vi "Calculate Vertex Array.vi"(8 "error in (no error)":errorcluster, 9 "Coordinates System":enum16{"Cartesian", "Cylindrical", "Spherical"}(ring)=enum."Spherical", 10 "3D Waterfall Datatype.lvclass in":refnum<class "3D Waterfall Datatype.lvclass">, 11 "Plot Representation In":T1) -> (0 "error out":errorcluster, 1 "Dup Coordinates System":enum16{"Cartesian", "Cylindrical", "Spherical"}(ring)=enum."Spherical", 2 "3D Waterfall Datatype.lvclass out":refnum<class "3D Waterfall Datatype.lvclass">, 3 "Plot Representation Out":T1)   [LabVIEW 2020, in "3D Waterfall Datatype.lvclass"]
uses:
  <vilib>/Math Plots/3D Math Plots/3D Waterfall/3D Waterfall Datatype/3D Waterfall Datatype.lvclass
  <vilib>/Math Plots/3D Math Plots/3D Plot/3D Plot/Typedef/Plot Representation.ctl
  <vilib>/Math Plots/3D Math Plots/3D Plot/3D Plot/Typedef/Range Clusters.ctl
  <vilib>/Math Plots/3D Math Plots/3D Plot/3D Plot/Typedef/Mesh Data.ctl
  <vilib>/Math Plots/3D Math Plots/3D Waterfall/3D Waterfall Datatype/3D Waterfall Datatype.lvclass/3D Waterfall Datatype.ctl
  <vilib>/Math Plots/3D Math Plots/3D Plot/3D Plot Datatype/3D Plot Datatype.lvclass
  <vilib>/Math Plots/3D Math Plots/3D Plot/3D Plot/3D Plot.lvclass
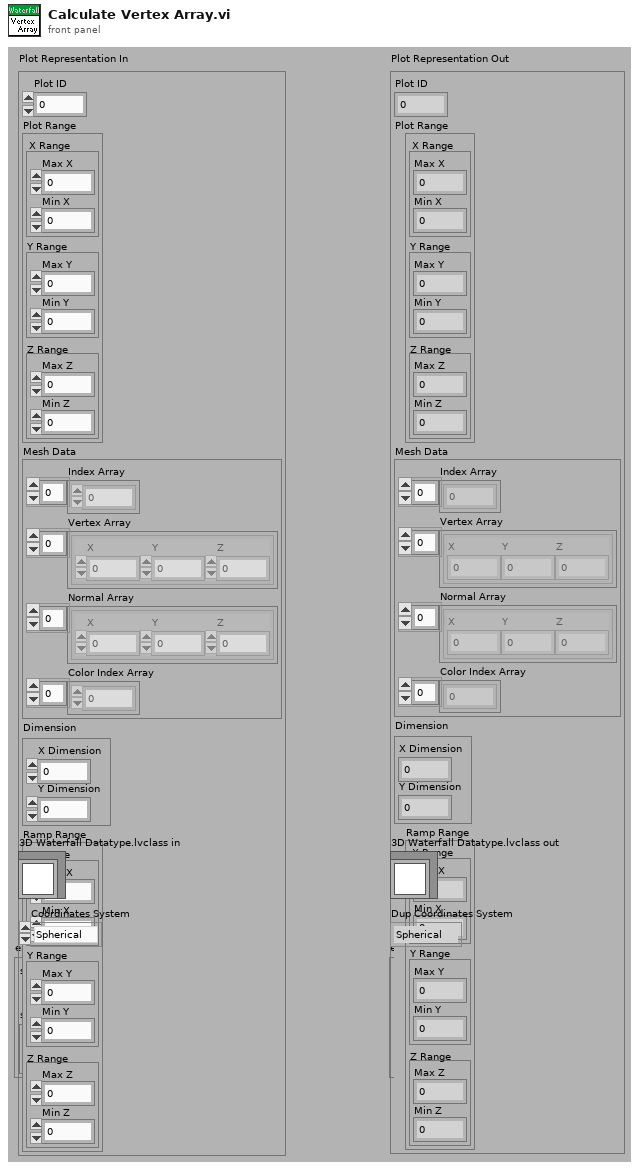
[diagram p1: front panel]
types:
  T1 = typedef "3D Plot.lvclass/Plot Representation.ctl" = cluster{"Plot ID":i32, "Plot Range":T2, "Mesh Data":T3, "Dimension":cluster{"X Dimension":i32, "Y Dimension":i32}, "Ramp Range":T2}
  T2 = typedef "3D Plot.lvclass/Range Clusters.ctl" = cluster{"X Range":cluster{"Max X":sgl, "Min X":sgl}, "Y Range":cluster{"Max Y":sgl, "Min Y":sgl}, "Z Range":cluster{"Max Z":sgl, "Min Z":sgl}}
  T3 = typedef "3D Plot.lvclass/Mesh Data.ctl" = cluster{"Index Array":u32[], "Vertex Array":cluster{"X":sgl, "Y":sgl, "Z":sgl}[], "Normal Array":cluster{"X":sgl, "Y":sgl, "Z":sgl}[], "Color Index Array":i32[]}
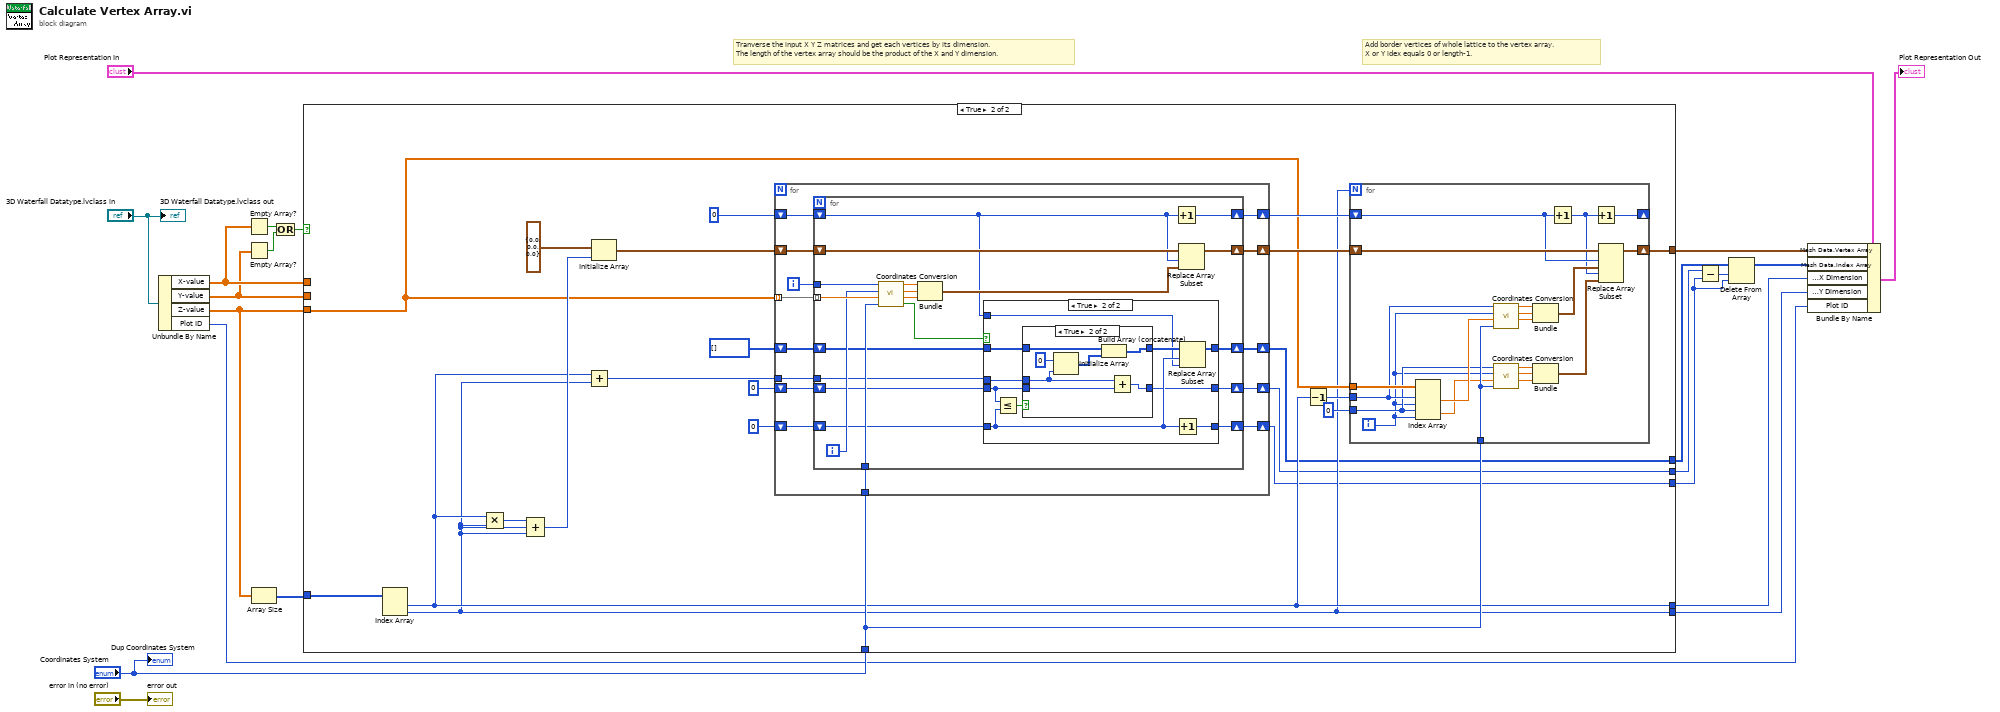
[diagram p0: block diagram]
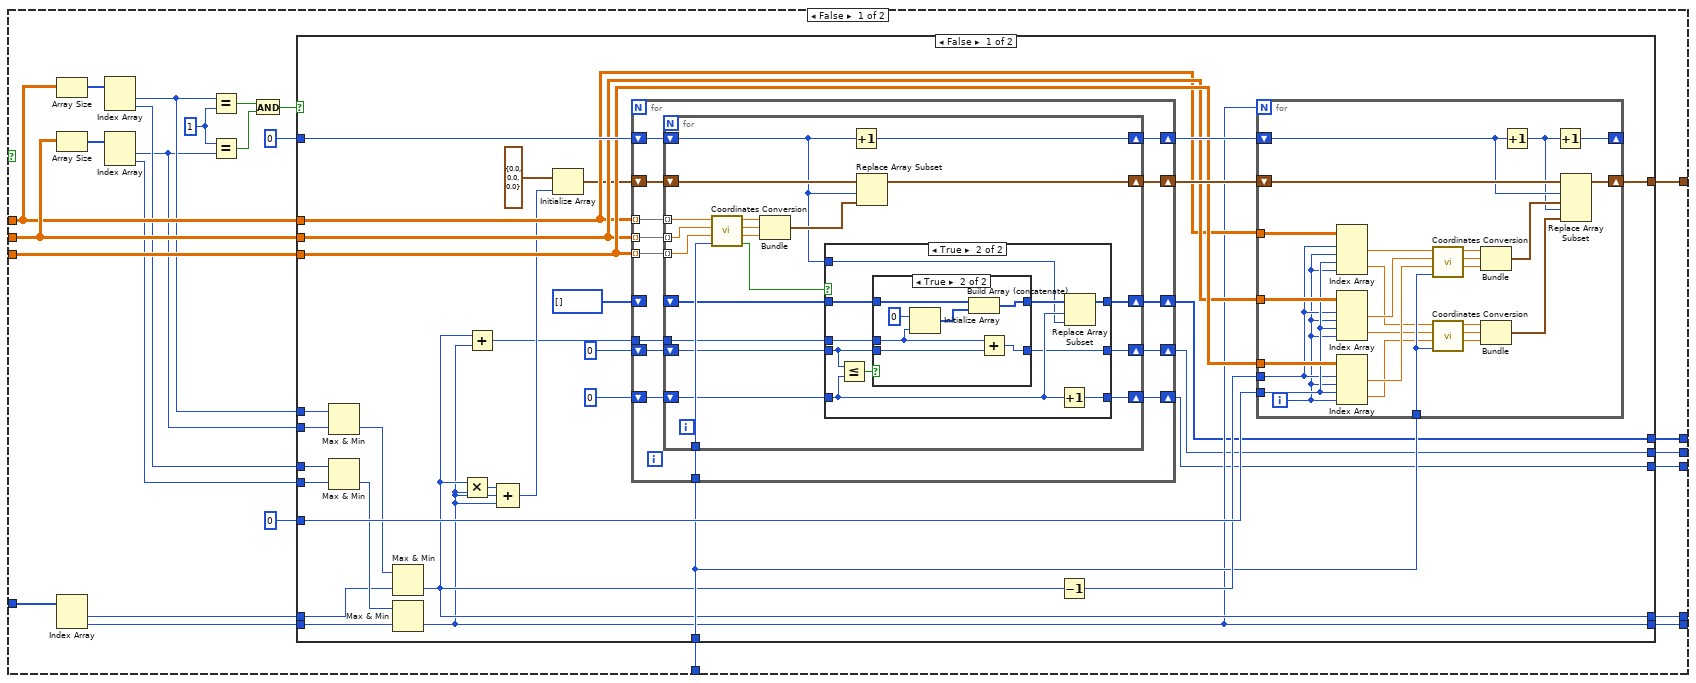
[diagram p2: hidden frame]
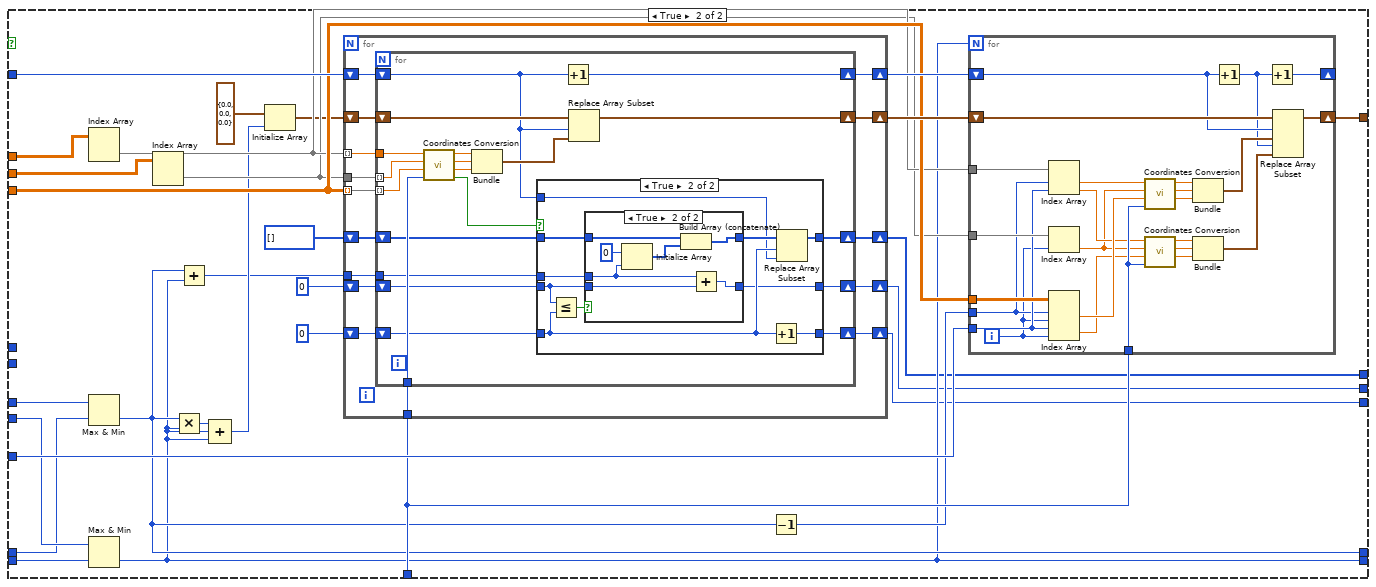
[diagram p5: hidden frame]
diagram:
  # "Add border vertices of whole lattice to the vertex array.\nX or Y idex equals 0 or length-1."
  # "Tranverse the input X Y Z matrices and get each vertices by its dimension.\nThe length of the vertex array should be the product of the X and Y dimension."
  n1 = Unbundle By Name("3D Waterfall Datatype.lvclass in") -> ("X-value"=w7:sgl[][], "Y-value"=w6:sgl[][], "Z-value"=w11:sgl[][], "Plot ID"=w14:i32)
  n2 = Empty Array?(array=w7) -> (empty?=w10:bool)
  n3 = Empty Array?(array=w6) -> (empty?=w9:bool)
  n4 = Array Size(array=w11) -> (size(s)=w16:i32[])
  n5 = Or(x=w10, y=w9) -> (x .or. y?=w8:bool)
  n6 = case shown="True" w8 {
    tunnel: "Coordinates System" -> [w33 w292]
    tunnel: w6 -> [w35 _]
    tunnel: w7 -> [w34 _]
    tunnel: w16 -> [w38 w286]
    tunnel: [w37 w284] -> w15
    tunnel: [w27 w275] -> w13
    tunnel: [w28 w276] -> w12
    tunnel: w11 -> [w39 w280]
    tunnel: [w24 w273] -> w4
    tunnel: [w23 w272] -> w2
    tunnel: [w22 w271] -> w1
    frame False {
      w42 = 1 ("x")
      n7 = Array Size(array=w34) -> (size(s)=w40:i32[])
      n8 = Array Size(array=w35) -> (size(s)=w41:i32[])
      n9 = Index Array(array=w38) -> (element #1=w30:i32, element #2=w32:i32)  [unwired: 2 in]
      n10 = Index Array(array=w40) -> (element #1=w26:i32, element #2=w29:i32)  [unwired: 2 in]
      n11 = Index Array(array=w41) -> (element #1=w25:i32, element #2=w31:i32)  [unwired: 2 in]
      n12 = Equal?(x=w26, y=w42) -> (x = y?=w43:bool)
      n13 = Equal?(x=w42, y=w25) -> (x = y?=w44:bool)
      n14 = And(x=w43, y=w44) -> (x .and. y?=w36:bool)
      n15 = case shown="False" w36 {
        tunnel: 0 -> [w75 w188]
        tunnel: 0 -> [w74 w186]
        tunnel: w39 -> [w72 w181]
        tunnel: [w73 w184] -> w37
        tunnel: w35 -> [w71 w182]
        tunnel: w34 -> [w70 w183]
        tunnel: w33 -> [w56 w177]
        tunnel: w32 -> [w58 w172]
        tunnel: w31 -> [w60 w171]
        tunnel: w30 -> [w57 w170]
        tunnel: w29 -> [w61 w169]
        tunnel: [w52 w165] -> w28
        tunnel: [w51 w164] -> w27
        tunnel: w26 -> [w64 _]
        tunnel: w25 -> [w63 _]
        tunnel: [w49 w162] -> w24
        tunnel: [w48 w161] -> w23
        tunnel: [w47 w160] -> w22
        frame False {
          n16 = Max & Min(x=w64, y=w63) -> (min(x,y)=w62:i32)  [unwired: 1 out]
          n17 = Max & Min(x=w61, y=w60) -> (min(x,y)=w59:i32)  [unwired: 1 out]
          n18 = Max & Min(x=w62, y=w57) -> (min(x,y)=w52:i32)  [unwired: 1 out]
          n19 = Max & Min(x=w59, y=w58) -> (min(x,y)=w51:i32)  [unwired: 1 out]
          n20 = Multiply(x=w52, y=w51) -> (x*y=w69:i32)
          n21 = Add(x=w52, y=w51) -> (x+y=w50:i32)
          n22 = Compound Arithmetic op=ADD(w69, w51, w51) -> (w67:i32)
          n23 = Initialize Array(cluster{"X":sgl, "Y":sgl, "Z":sgl} {"X"=0.0, "Y"=0.0, "Z"=0.0} ("3D Point"), w67) -> (w66:cluster{"X":sgl, "Y":sgl, "Z":sgl}[])
          n24 = for {
            shift-right: [w116] -> w76
            shift-left: w66 -> [w117]
            tunnel: w72 -> [w115] mode=indexing
            tunnel: w70 -> [w113] mode=indexing
            tunnel: w71 -> [w114] mode=indexing
            tunnel: w56 -> [w112]
            shift-right: [w110] -> w77
            shift-left: w75 -> [w111]
            shift-right: [w107] -> w47
            shift-left: 0 -> [w106]
            shift-right: [w108] -> w48
            shift-left: 0 -> [w105]
            shift-right: [w109] -> w49
            shift-left: u32[] [] -> [_]
            tunnel: w50 -> [w104]
            n25 = for {
              tunnel: w115 -> [w133] mode=indexing
              shift-right: [w137] -> w116
              shift-left: w117 -> [w136]
              tunnel: w114 -> [w134] mode=indexing
              tunnel: w113 -> [w135] mode=indexing
              tunnel: w112 -> [w129]
              shift-right: [w127] -> w110
              shift-left: w111 -> [w125]
              shift-right: [w122] -> w107
              shift-left: w106 -> [w119]
              shift-right: [w123] -> w108
              shift-left: w105 -> [w120]
              shift-right: [w124] -> w109
              shift-left: _ -> [w121]
              tunnel: w104 -> [w118]
              n26 = call <vilib>:"Coordinates Conversion.vi"("Coordinates System"=w129, "Z in"=w133, "Y in"=w134, "X in"=w135) -> ("NaN?"=w126:bool, "Z out"=w130:sgl, "Y out"=w131:sgl, "X out"=w132:sgl)  [unwired: 4 out]
              n27 = Bundle("X out"=w132, "Y out"=w131, "Z out"=w130) -> (w128:cluster{"X out":sgl, "Y out":sgl, "Z out":sgl})  [unwired: 1 out]
              n28 = case shown="True" w126 {
                tunnel: w121 -> [w140 w148]
                tunnel: [w140 w144] -> w124
                tunnel: w125 -> [_ w145]
                tunnel: w119 -> [w139 w146]
                tunnel: [w139 w150] -> w122
                tunnel: w120 -> [w138 w142]
                tunnel: [w138 w143] -> w123
                tunnel: w118 -> [_ w141]
                frame False {
                }
                frame True {
                  n29 = Less Or Equal?(x=w142, y=w146) -> (x <= y?=w149:bool)
                  n30 = case shown="True" w149 {
                    tunnel: w148 -> [w152 w159]
                    tunnel: [w152 w158] -> w147
                    tunnel: [w151 w154] -> w143
                    tunnel: w142 -> [w151 w155]
                    tunnel: w141 -> [_ w153]
                    frame False {
                    }
                    frame True {
                      n31 = Initialize Array(u32 0, w153) -> (w156:u32[])
                      n32 = Build Array (concatenate)(w159, w156) -> (w158:u32[])
                      n33 = Add(x=w153, y=w155) -> (x+y=w154:i32)
                    }
                  }
                  n34 = Increment(x=w146) -> (x+1=w150:i32)
                  n35 = Replace Array Subset(array=w147, new element=w145, index=w146) -> (w144:u32[])
                }
              }
              n36 = Increment(x=w125) -> (x+1=w127:i32)
              n37 = Replace Array Subset(array=w136, new element=w128, index=w125) -> (w137:cluster{"X":sgl, "Y":sgl, "Z":sgl}[])
            }
          }
          n38 = Decrement(x=w52) -> (x-1=w65:i32)
          n39 = for {
            N: w51 -> [_]
            shift-right: [w99] -> w73
            shift-left: w76 -> [w100]
            tunnel: w72 -> [w101]
            tunnel: w70 -> [w103]
            tunnel: w71 -> [w102]
            tunnel: w65 -> [w97]
            tunnel: w74 -> [w98]
            tunnel: w56 -> [w96]
            shift-right: [w78] -> _
            shift-left: w77 -> [w80]
            i -> [w83]
            n40 = Index Array(array=w103, index (row) #1=w97, index (col) #1=w83, index (row) #2=w98, index (col) #2=w83) -> (element #1=w95:sgl, element #2=w89:sgl)
            n41 = Index Array(array=w102, index (row) #1=w97, index (col) #1=w83, index (row) #2=w98, index (col) #2=w83) -> (element #1=w94:sgl, element #2=w88:sgl)
            n42 = Index Array(array=w101, index (row) #1=w97, index (col) #1=w83, index (row) #2=w98, index (col) #2=w83) -> (element #1=w93:sgl, element #2=w87:sgl)
            n43 = call <vilib>:"Coordinates Conversion.vi"("Coordinates System"=w96, "Z in"=w93, "Y in"=w94, "X in"=w95) -> ("Z out"=w92:sgl, "Y out"=w91:sgl, "X out"=w90:sgl)  [unwired: 5 out]
            n44 = call <vilib>:"Coordinates Conversion.vi"("Coordinates System"=w96, "Z in"=w87, "Y in"=w88, "X in"=w89) -> ("Z out"=w84:sgl, "Y out"=w85:sgl, "X out"=w86:sgl)  [unwired: 5 out]
            n45 = Bundle("X out"=w90, "Y out"=w91, "Z out"=w92) -> (w81:cluster{"X out":sgl, "Y out":sgl, "Z out":sgl})  [unwired: 1 out]
            n46 = Bundle("X out"=w86, "Y out"=w85, "Z out"=w84) -> (w82:cluster{"X out":sgl, "Y out":sgl, "Z out":sgl})  [unwired: 1 out]
            n47 = Increment(x=w80) -> (x+1=w79:i32)
            n48 = Increment(x=w79) -> (x+1=w78:i32)
            n49 = Replace Array Subset(array=w100, new element #1=w81, index #1=w80, new element #2=w82, index #2=w79) -> (w99:cluster{"X":sgl, "Y":sgl, "Z":sgl}[])
          }
        }
        frame True {
          n50 = Index Array(array=w183) -> (element=w180:sgl[])  [unwired: 2 in]
          n51 = Max & Min(x=w169, y=w170) -> (min(x,y)=w165:i32)  [unwired: 1 out]
          n52 = Max & Min(x=w171, y=w172) -> (min(x,y)=w164:i32)  [unwired: 1 out]
          n53 = Index Array(array=w182) -> (element=w179:sgl[])  [unwired: 2 in]
          n54 = Multiply(x=w165, y=w164) -> (x*y=w178:i32)
          n55 = Add(x=w165, y=w164) -> (x+y=w163:i32)
          n56 = Compound Arithmetic op=ADD(w178, w164, w164) -> (w175:i32)
          n57 = Initialize Array(cluster{"X":sgl, "Y":sgl, "Z":sgl} {"X"=0.0, "Y"=0.0, "Z"=0.0} ("3D Point"), w175) -> (w174:cluster{"X":sgl, "Y":sgl, "Z":sgl}[])
          n58 = for {
            shift-right: [w227] -> w185
            shift-left: w174 -> [w228]
            tunnel: w181 -> [w226] mode=indexing
            tunnel: w180 -> [w224] mode=indexing
            tunnel: w179 -> [w225]
            tunnel: w177 -> [w223]
            shift-right: [w221] -> w187
            shift-left: w188 -> [w222]
            shift-right: [w220] -> w162
            shift-left: u32[] [] -> [w215]
            shift-right: [w219] -> w161
            shift-left: 0 -> [w217]
            shift-right: [w218] -> w160
            shift-left: 0 -> [w216]
            tunnel: w163 -> [w214]
            n59 = for {
              tunnel: w226 -> [w244] mode=indexing
              shift-right: [w248] -> w227
              shift-left: w228 -> [w247]
              tunnel: w225 -> [w245] mode=indexing
              tunnel: w224 -> [w246]
              tunnel: w223 -> [w240]
              shift-right: [w238] -> w221
              shift-left: w222 -> [w231]
              shift-right: [w237] -> w220
              shift-left: w215 -> [w232]
              shift-right: [w236] -> w219
              shift-left: w217 -> [w233]
              shift-right: [w235] -> w218
              shift-left: w216 -> [w234]
              tunnel: w214 -> [w229]
              n60 = call <vilib>:"Coordinates Conversion.vi"("Coordinates System"=w240, "Z in"=w244, "Y in"=w245, "X in"=w246) -> ("NaN?"=w230:bool, "Z out"=w241:sgl, "Y out"=w242:sgl, "X out"=w243:sgl)  [unwired: 4 out]
              n61 = Bundle("X out"=w243, "Y out"=w242, "Z out"=w241) -> (w239:cluster{"X out":sgl, "Y out":sgl, "Z out":sgl})  [unwired: 1 out]
              n62 = case shown="True" w230 {
                tunnel: w232 -> [w251 w259]
                tunnel: [w251 w255] -> w237
                tunnel: w231 -> [_ w256]
                tunnel: w234 -> [w250 w257]
                tunnel: [w250 w261] -> w235
                tunnel: w233 -> [w249 w253]
                tunnel: [w249 w254] -> w236
                tunnel: w229 -> [_ w252]
                frame False {
                }
                frame True {
                  n63 = Less Or Equal?(x=w253, y=w257) -> (x <= y?=w260:bool)
                  n64 = case shown="True" w260 {
                    tunnel: w259 -> [w263 w270]
                    tunnel: [w263 w269] -> w258
                    tunnel: [w262 w265] -> w254
                    tunnel: w253 -> [w262 w266]
                    tunnel: w252 -> [_ w264]
                    frame False {
                    }
                    frame True {
                      n65 = Initialize Array(u32 0, w264) -> (w267:u32[])
                      n66 = Build Array (concatenate)(w270, w267) -> (w269:u32[])
                      n67 = Add(x=w264, y=w266) -> (x+y=w265:i32)
                    }
                  }
                  n68 = Increment(x=w257) -> (x+1=w261:i32)
                  n69 = Replace Array Subset(array=w258, new element=w256, index=w257) -> (w255:u32[])
                }
              }
              n70 = Increment(x=w231) -> (x+1=w238:i32)
              n71 = Replace Array Subset(array=w247, new element=w239, index=w231) -> (w248:cluster{"X":sgl, "Y":sgl, "Z":sgl}[])
            }
          }
          n72 = Decrement(x=w165) -> (x-1=w173:i32)
          n73 = for {
            N: w164 -> [_]
            shift-right: [w209] -> w184
            shift-left: w185 -> [w210]
            tunnel: w181 -> [w211]
            tunnel: w180 -> [w213]
            tunnel: w179 -> [w212]
            tunnel: w173 -> [w207]
            tunnel: w186 -> [w208]
            tunnel: w177 -> [w206]
            shift-right: [w191] -> _
            shift-left: w187 -> [w193]
            i -> [w189]
            n74 = Index Array(array=w213, index #1=w207, index #2=w208) -> (element #1=w205:sgl, element #2=w200:sgl)
            n75 = Index Array(array=w212, index=w189) -> (element=w190:sgl)
            n76 = Index Array(array=w211, index (row) #1=w207, index (col) #1=w189, index (row) #2=w208, index (col) #2=w189) -> (element #1=w204:sgl, element #2=w199:sgl)
            n77 = call <vilib>:"Coordinates Conversion.vi"("Coordinates System"=w206, "Z in"=w204, "Y in"=w190, "X in"=w205) -> ("Z out"=w203:sgl, "Y out"=w202:sgl, "X out"=w201:sgl)  [unwired: 5 out]
            n78 = call <vilib>:"Coordinates Conversion.vi"("Coordinates System"=w206, "Z in"=w199, "Y in"=w190, "X in"=w200) -> ("Z out"=w196:sgl, "Y out"=w197:sgl, "X out"=w198:sgl)  [unwired: 5 out]
            n79 = Bundle("X out"=w201, "Y out"=w202, "Z out"=w203) -> (w194:cluster{"X out":sgl, "Y out":sgl, "Z out":sgl})  [unwired: 1 out]
            n80 = Bundle("X out"=w198, "Y out"=w197, "Z out"=w196) -> (w195:cluster{"X out":sgl, "Y out":sgl, "Z out":sgl})  [unwired: 1 out]
            n81 = Increment(x=w193) -> (x+1=w192:i32)
            n82 = Increment(x=w192) -> (x+1=w191:i32)
            n83 = Replace Array Subset(array=w210, new element #1=w194, index #1=w193, new element #2=w195, index #2=w192) -> (w209:cluster{"X":sgl, "Y":sgl, "Z":sgl}[])
          }
        }
      }
    }
    frame True {
      n84 = Index Array(array=w286) -> (element #1=w276:i32, element #2=w275:i32)  [unwired: 2 in]
      n85 = Multiply(x=w276, y=w275) -> (x*y=w290:i32)
      n86 = Compound Arithmetic op=ADD(w290, w275, w275) -> (w291:i32)
      n87 = Add(x=w276, y=w275) -> (x+y=w277:i32)
      n88 = Initialize Array(cluster{"X":sgl, "Y":sgl, "Z":sgl} {"X"=0.0, "Y"=0.0, "Z"=0.0} ("3D Point"), w291) -> (w288:cluster{"X":sgl, "Y":sgl, "Z":sgl}[])
      n89 = for {
        shift-right: [w325] -> w281
        shift-left: w288 -> [w326]
        tunnel: w280 -> [w324] mode=indexing
        tunnel: w292 -> [w323]
        shift-right: [w321] -> w283
        shift-left: 0 -> [w322]
        shift-right: [w319] -> w273
        shift-left: u32[] [] -> [w316]
        shift-right: [w318] -> w272
        shift-left: 0 -> [w314]
        shift-right: [w317] -> w271
        shift-left: 0 -> [w315]
        tunnel: w277 -> [w313]
        i -> [w320]
        n90 = for {
          tunnel: w324 -> [w343] mode=indexing
          shift-right: [w346] -> w325
          shift-left: w326 -> [w345]
          tunnel: w320 -> [w344]
          tunnel: w323 -> [w339]
          shift-right: [w337] -> w321
          shift-left: w322 -> [w330]
          shift-right: [w333] -> w317
          shift-left: w315 -> [w329]
          shift-right: [w334] -> w318
          shift-left: w314 -> [w328]
          shift-right: [w335] -> w319
          shift-left: w316 -> [w332]
          tunnel: w313 -> [w327]
          i -> [w336]
          n91 = call <vilib>:"Coordinates Conversion.vi"("Coordinates System"=w339, "Z in"=w343, "Y in"=w336, "X in"=w344) -> ("NaN?"=w331:bool, "Z out"=w340:sgl, "Y out"=w341:sgl, "X out"=w342:sgl)  [unwired: 4 out]
          n92 = Bundle("X out"=w342, "Y out"=w341, "Z out"=w340) -> (w338:cluster{"X out":sgl, "Y out":sgl, "Z out":sgl})  [unwired: 1 out]
          n93 = case shown="True" w331 {
            tunnel: w332 -> [w349 w357]
            tunnel: [w349 w353] -> w335
            tunnel: w330 -> [_ w354]
            tunnel: w329 -> [w348 w355]
            tunnel: [w348 w359] -> w333
            tunnel: w328 -> [w347 w351]
            tunnel: [w347 w352] -> w334
            tunnel: w327 -> [_ w350]
            frame False {
            }
            frame True {
              n94 = Less Or Equal?(x=w351, y=w355) -> (x <= y?=w358:bool)
              n95 = case shown="True" w358 {
                tunnel: w357 -> [w361 w368]
                tunnel: [w361 w367] -> w356
                tunnel: [w360 w363] -> w352
                tunnel: w351 -> [w360 w364]
                tunnel: w350 -> [_ w362]
                frame False {
                }
                frame True {
                  n96 = Initialize Array(u32 0, w362) -> (w365:u32[])
                  n97 = Build Array (concatenate)(w368, w365) -> (w367:u32[])
                  n98 = Add(x=w362, y=w364) -> (x+y=w363:i32)
                }
              }
              n99 = Increment(x=w355) -> (x+1=w359:i32)
              n100 = Replace Array Subset(array=w356, new element=w354, index=w355) -> (w353:u32[])
            }
          }
          n101 = Increment(x=w330) -> (x+1=w337:i32)
          n102 = Replace Array Subset(array=w345, new element=w338, index=w330) -> (w346:cluster{"X":sgl, "Y":sgl, "Z":sgl}[])
        }
      }
      n103 = Decrement(x=w276) -> (x-1=w285:i32)
      n104 = for {
        N: w275 -> [_]
        shift-right: [w310] -> w284
        shift-left: w281 -> [w311]
        tunnel: w280 -> [w312]
        tunnel: w285 -> [w295]
        tunnel: 0 -> [w294]
        tunnel: w292 -> [w309]
        shift-right: [w296] -> _
        shift-left: w283 -> [w298]
        i -> [w293]
        n105 = Index Array(array=w312, index (row) #1=w295, index (col) #1=w293, index (row) #2=w294, index (col) #2=w293) -> (element #1=w308:sgl, element #2=w304:sgl)
        n106 = call <vilib>:"Coordinates Conversion.vi"("Coordinates System"=w309, "Z in"=w308, "Y in"=w293, "X in"=w295) -> ("Z out"=w307:sgl, "Y out"=w306:sgl, "X out"=w305:sgl)  [unwired: 5 out]
        n107 = call <vilib>:"Coordinates Conversion.vi"("Coordinates System"=w309, "Z in"=w304, "Y in"=w293, "X in"=w294) -> ("Z out"=w301:sgl, "Y out"=w302:sgl, "X out"=w303:sgl)  [unwired: 5 out]
        n108 = Bundle("X out"=w305, "Y out"=w306, "Z out"=w307) -> (w299:cluster{"X out":sgl, "Y out":sgl, "Z out":sgl})  [unwired: 1 out]
        n109 = Bundle("X out"=w303, "Y out"=w302, "Z out"=w301) -> (w300:cluster{"X out":sgl, "Y out":sgl, "Z out":sgl})  [unwired: 1 out]
        n110 = Increment(x=w298) -> (x+1=w297:i32)
        n111 = Increment(x=w297) -> (x+1=w296:i32)
        n112 = Replace Array Subset(array=w311, new element #1=w299, index #1=w298, new element #2=w300, index #2=w297) -> (w310:cluster{"X":sgl, "Y":sgl, "Z":sgl}[])
      }
    }
  }
  n113 = Subtract(x=w2, y=w1) -> (x-y=w5:i32)
  n114 = Delete From Array(array=w4, length=w5, index=w1) -> (array with subset deleted=w3:u32[])  [unwired: 1 out]
  n115 = Bundle By Name(cluster="Plot Representation In", "Mesh Data.Vertex Array"=w15, "Mesh Data.Index Array"=w3, "Dimension.X Dimension"=w12, "Dimension.Y Dimension"=w13, "Plot ID"=w14) -> (→"Plot Representation Out":T1)
  "error out" <- "error in (no error)"
  "3D Waterfall Datatype.lvclass out" <- "3D Waterfall Datatype.lvclass in"
  "Dup Coordinates System" <- "Coordinates System"
